vi "Convert Signal Parameters String to Cluster.vi"(8 "error in (no error)":errorcluster, 11 "Signal Parameters":string[](array[string])) -> (0 "error out":errorcluster, 3 "Signal Parameters":T1 {"Byte Order" items=["Little Endian", "Big Endian"]; "Data Type" items=["Signed", "Unsigned", "IEEE Float"]})   [LabVIEW 2015, in "Diagnostics Addon System Explorer.lvlib"]
uses:
  Diagnostics Addon System Explorer.lvlib
  Shared/Signal Parameters.ctl
  Shared/Diagnostics Addon Shared.lvlib
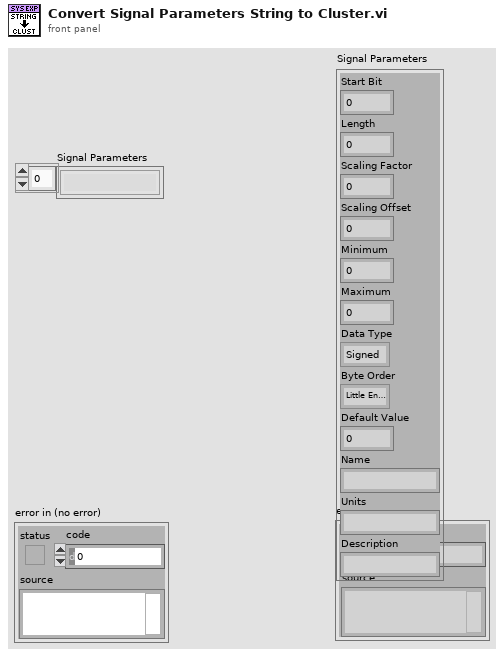
[diagram p1: front panel]
types:
  T1 = typedef "Diagnostics Addon Shared.lvlib/Signal Parameters.ctl" = cluster{"Start Bit":u8, "Length":u8, "Scaling Factor":dbl, "Scaling Offset":dbl, "Minimum":dbl, "Maximum":dbl, "Data Type":u32, "Byte Order":u32, "Default Value":dbl, "Name":string, "Units":string, "Description":string}
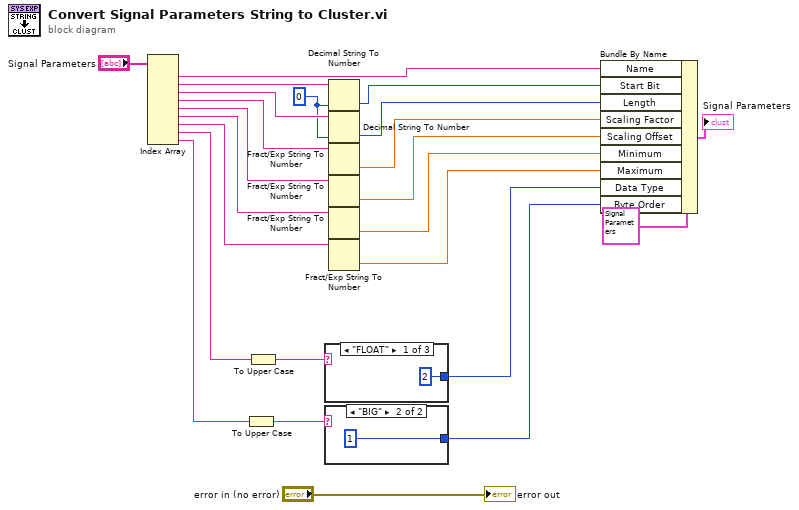
[diagram p0: block diagram]
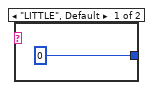
[diagram p2: hidden frame]
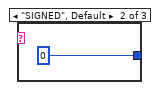
[diagram p3: hidden frame]
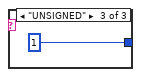
[diagram p4: hidden frame]
diagram:
  w18 = u8 0 ("Start Bit")
  n1 = Index Array(array="Signal Parameters") -> (element #1=w21:string, element #2=w20:string, element #3=w19:string, element #4=w15:string, element #5=w14:string, element #6=w13:string, element #7=w12:string, element #8=w6:string, element #9=w3:string)  [unwired: 9 in]
  n2 = To Upper Case(1:w3) -> (0:w2:string)
  n3 = To Upper Case(1:w6) -> (0:w5:string)
  n4 = case shown="\"FLOAT\"" w5 {
    tunnel: [2 0 1] -> w4
    frame "FLOAT" {
    }
    frame "SIGNED", Default {
    }
    frame "UNSIGNED" {
    }
  }
  n5 = case shown="\"BIG\"" w2 {
    tunnel: [0 1] -> w1
    frame "LITTLE", Default {
    }
    frame "BIG" {
    }
  }
  n6 = Decimal String To Number(string=w20, default (0L)=w18) -> (number=w17:u8)  [unwired: 1 in, 1 out]
  n7 = Decimal String To Number(string=w19, default (0L)=w18) -> (number=w16:u8)  [unwired: 1 in, 1 out]
  n8 = Fract/Exp String To Number(string=w15) -> (number=w11:dbl)  [unwired: 3 in, 1 out]
  n9 = Fract/Exp String To Number(string=w14) -> (number=w10:dbl)  [unwired: 3 in, 1 out]
  n10 = Fract/Exp String To Number(string=w13) -> (number=w9:dbl)  [unwired: 3 in, 1 out]
  n11 = Fract/Exp String To Number(string=w12) -> (number=w8:dbl)  [unwired: 3 in, 1 out]
  n12 = Bundle By Name(cluster=T1 {"Start Bit"=0, "Length"=0, "Scaling Factor"=0.0, "Scaling Offset"=0.0, "Minimum"=0.0, "Maximum"=0.0, "Data Type"=0, "Byte Order"=0, "Default Value"=0.0, "Name"="", "Units"="", "Description"=""} ("Signal Parameters"), "Name"=w21, "Start Bit"=w17, "Length"=w16, "Scaling Factor"=w11, "Scaling Offset"=w10, "Minimum"=w9, "Maximum"=w8, "Data Type"=w4, "Byte Order"=w1) -> (→"Signal Parameters":T1)
  "error out" <- "error in (no error)"
